vi "Create Error Log.vi"(8 "Error In":errorcluster, 9 "Module Init Timestamp":timestamp, 10 "Application Name":string, 11 "The folder to store the Error Logs":path) -> (0 "Error Out":errorcluster, 3 "Full file path of the Error Log":path)   [LabVIEW 2023, in "Error Manager.lvlib" / "Error Log.lvclass"]
doc: "This VI creates the Error Log file"
uses:
  Error Log.lvclass
  Error Log Ref (class variable).vi
panel:
  # "Input\nInputs to the VI"
  # "Development\nControls or indicators that are useful for development or testing, but which are not outputs of the VI."
  # "Output\nOutputs of the VI"
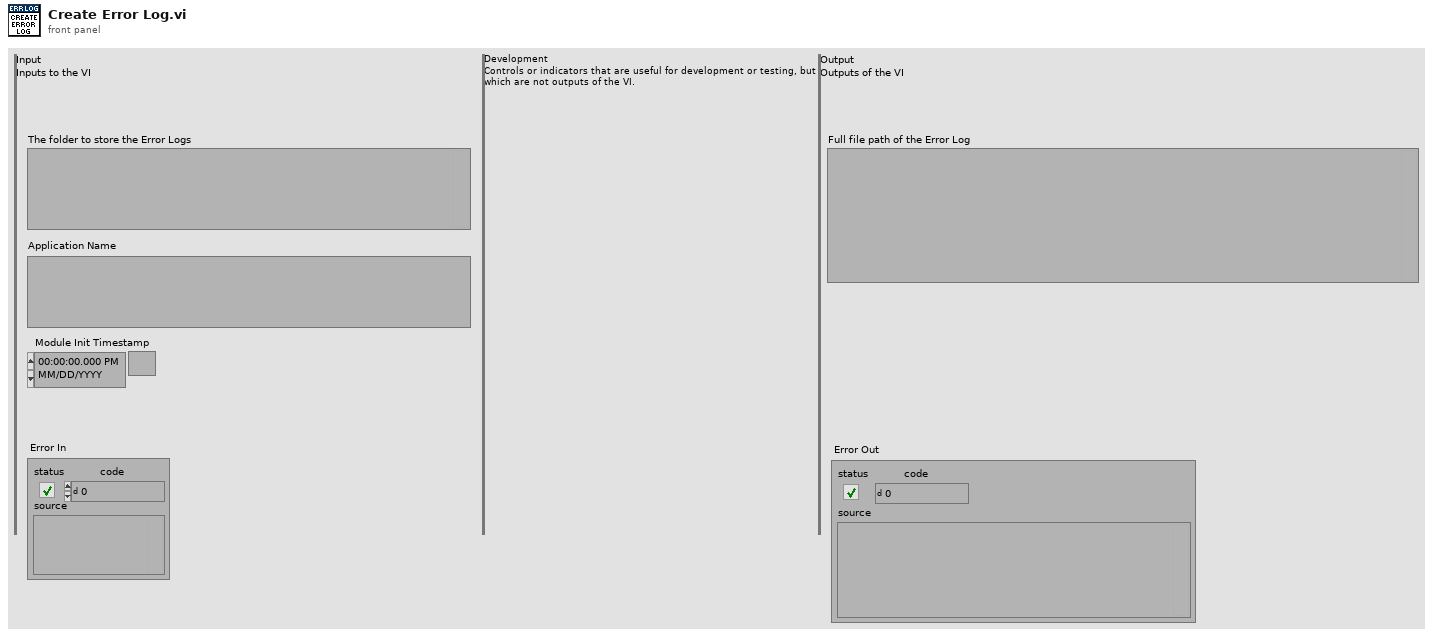
[diagram p1: front panel]
types:
  T1 = enum16{"open", "replace", "create", "open or create", "replace or create", "replace or create with confirmation"}
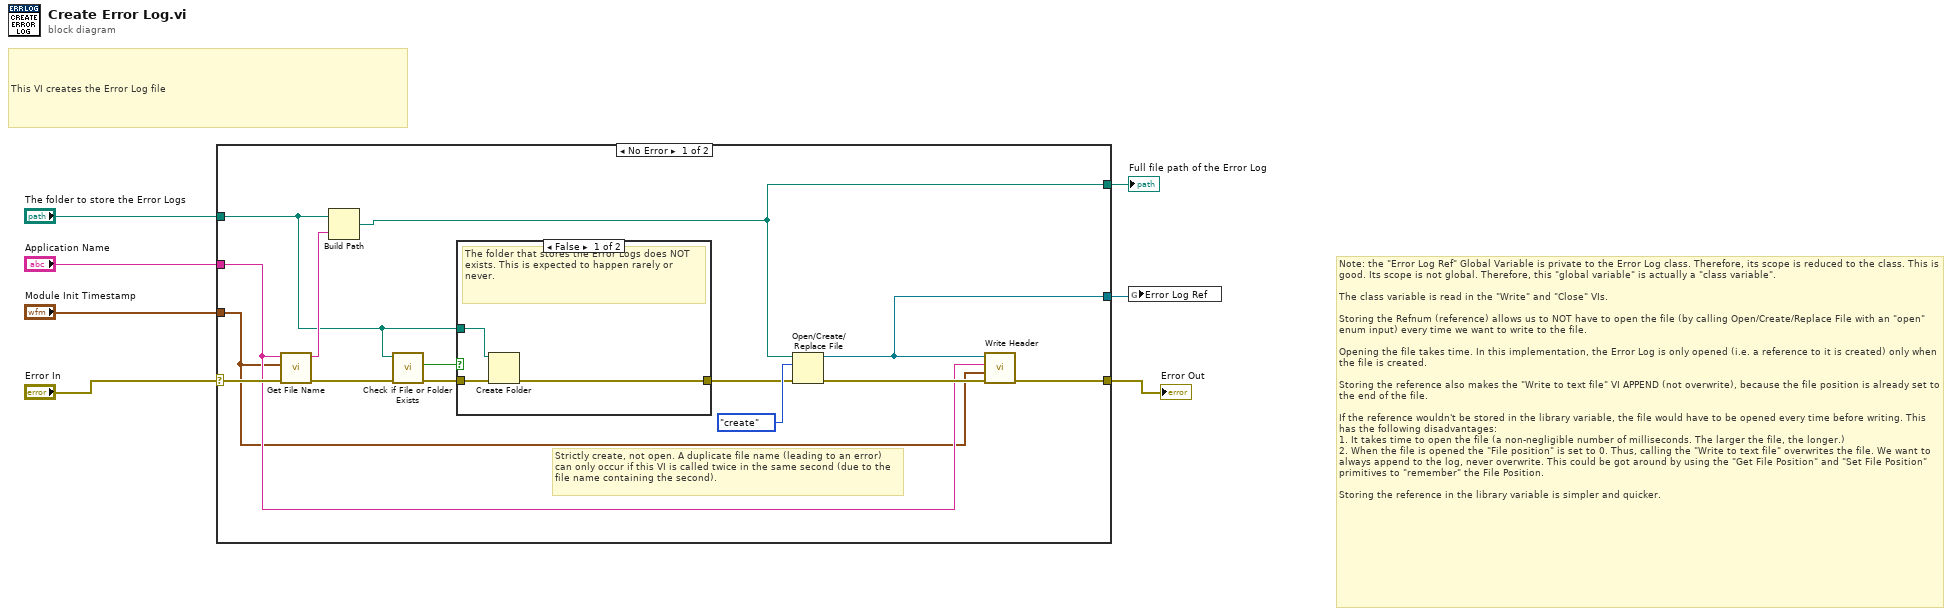
[diagram p0: block diagram]
diagram:
  # "This VI creates the Error Log file"
  # "Note: the \"Error Log Ref\" Global Variable is private to the Error Log class. Therefore, its scope is reduced to the class. This is good. Its scope is not global. Therefore, this \"global variable\" is actually a \"class variable\".\n\nThe class variable is read in the \"Write\" and \"Close\" VIs.\n\nStoring the Refnum (reference) allows us to NOT have to open the file (by calling Open/Create/Replace File with an \"open\" enum input) every time we want to write to the file.\n\nOpening the file takes time. In this implementation, the Error Log is only opened (i.e. a reference to it is created) only when the file is created.\n\nStoring the reference also makes the \"Write to text file\" VI APPEND (not overwrite), because the file position is already set to the end of the file. \n\nIf the reference wouldn't be stored in the library variable, the file would have to be opened every time before writing. This has the following disadvantages:\n1. It takes time to open the file (a non-negligible number of milliseconds. The larger the file, the longer.)\n2. When the file is opened the \"File position\" is set to 0. Thus, calling the \"Write to text file\" overwrites the file. We want to always append to the log, never overwrite. This could be got around by using the \"Get File Position\" and \"Set File Position\" primitives to \"remember\" the File Position.\n\nStoring the reference in the library variable is simpler and quicker."
  n1 = case shown="No Error" "Error In" {
    selector: "Error In" -> [w20 w26]
    tunnel: [w11 _] -> w6
    tunnel: [w12 _] -> w4
    tunnel: [w13 w26] -> w5
    tunnel: "The folder to store the Error Logs" -> [w10 _]
    tunnel: "Application Name" -> [w9 _]
    tunnel: "Module Init Timestamp" -> [w8 _]
    frame No Error {
      # "Strictly create, not open. A duplicate file name (leading to an error) can only occur if this VI is called twice in the same second (due to the file name containing the second)."
      n2 = call "Get File Name.vi"("error in (no error)"=w20, "Module Init Timestamp"=w8, "Application Name"=w9) -> ("error out"=w19:errorcluster, "Error Log Filename"=w15:string)  [unwired: 7 in]
      n3 = Build Path(base path=w10, name or relative path=w15) -> (appended path=w11:path)
      n4 = call <vilib>:"Check if File or Folder Exists.vi"("error in (no error)"=w19, "path"=w10) -> ("error out"=w18:errorcluster, "file or folder exists?"=w17:bool)  [unwired: 7 in, 1 out]
      n5 = case shown="False" w17 {
        tunnel: w18 -> [w24 w25]
        tunnel: w10 -> [w23 _]
        tunnel: [w22 w25] -> w16
        frame False {
          # "The folder that stores the Error Logs does NOT exists. This is expected to happen rarely or never."
          n6 = Create Folder(path (use dialog)=w23, error in=w24) -> (error out=w22:errorcluster)  [unwired: 1 in, 2 out]
        }
        frame True {
          # "Do nothing."
          # "The folder that stores the Error Logs already exists. Good. This is expected to happen most of the time."
        }
      }
      n7 = Open/Create/Replace File(file path (use dialog)=w11, error in=w16, operation (0:open)=T1."create") -> (refnum out=w12:refnum<file>, error out=w14:errorcluster)  [unwired: 3 in, 1 out]
      n8 = call "Write Header.vi"("error in (no error)"=w14, "Module Init Timestamp"=w8, "Application Name"=w9, "File refnum"=w12) -> ("error out"=w13:errorcluster)  [unwired: 7 in]
    }
    frame Error {
    }
  }
  "Error Out" <- w5
  "Full file path of the Error Log" <- w6
  n9 = global write "Error Log Ref (class variable).vi" "Error Log Ref"(w4) -> ()
